vi "test server.vi"   [LabVIEW 2012]
uses:
  <vilib>/Platform/TimedLoop/XDataNode/timing_clust.ctl
  <vilib>/Platform/TimedLoop/XDataNode/nitl_modes.ctl
  <vilib>/Platform/TimedLoop/XDataNode/wakeup.ctl
  <vilib>/Platform/TimedLoop/XDataNode/XDataNode.xnode
  <vilib>/Platform/TimedLoop/XDataNode/XDNodeRunTimeDep.lvlib
types:
  T1 = typedef "XDNodeRunTimeDep.lvlib/timing_clust.ctl" = cluster{"Expected End [f-1]":u64, "Actual End [f-1]":u64, "Finished Late? [f-1]":bool, "Expected End [i-1]":u64, "Actual End [i-1]":u64, "Finished Late? [i-1]":bool, "Expected Start [i]":u64, "Actual Start [i]":u64, "Expected Start [f]":u64, "Actual Start [f]":u64, "Source Name":string, "Structure Name":string, "Period":i64, "Deadline":i64, "Offset":i64, "Start":i64, "Priority":i32, "Timeout":i32, "Mode":T2, "Wakeup Reason":T3, "Error":errorcluster, "Source Type":string, "Secondary Source Type":string, "Global End Time":u64, "Global Start Time":u64, "Frame Duration":u64, "Iteration Duration":u64, "Assigned CPU":i32, "I/O Scan Engine Mode":u32}
  T2 = typedef "XDNodeRunTimeDep.lvlib/nitl_modes.ctl" = enum32{"No Change", "Process missed periods, maintain original phase", "Discard missed periods, maintain original phase", "Process missed periods, ignore original phase", "Discard missed periods, ignore original phase"}
  T3 = typedef "XDNodeRunTimeDep.lvlib/wakeup.ctl" = enum32{"Normal", "Aborted", "Asynchronous wakeup", "Timing source error", "Timed loop error", "Timeout"}
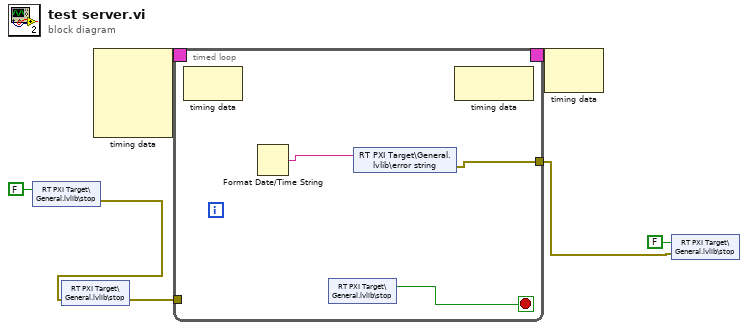
[diagram p0: block diagram]
diagram:
  n1 = shared-variable "RT PXI Target\\General.lvlib\\stop"(FALSE ("stop")) -> (error out=w6:errorcluster)  [unwired: 1 in]
  n2 = shared-variable "RT PXI Target\\General.lvlib\\stop"(error in=w6) -> (error out=w5:errorcluster)  [unwired: 1 out]
  n3 = node-c288() -> (w4:T1)  [unwired: 4 in]
  n4 = timed-loop {
    tunnel: w5 -> [_]
    timing: w4 -> [_]
    timing-out: [_] -> w3
    tunnel: [w8] -> w1
    stop <- w10 stop-if-true
    n5 = node-c288() -> ()  [unwired: 1 in, 1 out]
    n6 = Format Date/Time String() -> (date/time string=w9:string)  [unwired: 3 in]
    n7 = shared-variable "RT PXI Target\\General.lvlib\\stop"() -> (w10:bool)  [unwired: 1 in, 1 out]
    n8 = shared-variable "RT PXI Target\\General.lvlib\\error string"(w9) -> (error out=w8:errorcluster)  [unwired: 1 in]
    n9 = node-c288() -> ()  [unwired: 1 in, 1 out]
  }
  n10 = node-c288(w3) -> ()  [unwired: 1 out]
  n11 = shared-variable "RT PXI Target\\General.lvlib\\stop"(FALSE ("stop"), error in=w1) -> ()  [unwired: 1 out]
